vi "Run Process.vi"(8 "error in":errorcluster, 9 "Processes":cluster{"VI":refnum<vi>, "Parameters":variant}[](array[cluster]), 11 "VS Plugin Inline Async API in":refnum<class "VS Plugin Inline Async API.lvclass">) -> (0 "error out":errorcluster, 3 "VS Plugin Inline Async API out":refnum<class "VS Plugin Inline Async API.lvclass">)   [LabVIEW 2024, in "VS Plugin Inline Async API.lvlib" / "VS Plugin Inline Async API.lvclass"]
uses:
  VS Plugin Inline Async API.lvclass
  VS Plugin Inline Async API.lvclass/VS Plugin Inline Async API.ctl
  Process/Process.lvclass
  Process/Process.lvclass/Process.ctl
  Process/Write Name.vi
  Process/Write Process.Stop.vi
  Process/Write Process.Trigger.vi
  Process/Write Data Access.vi
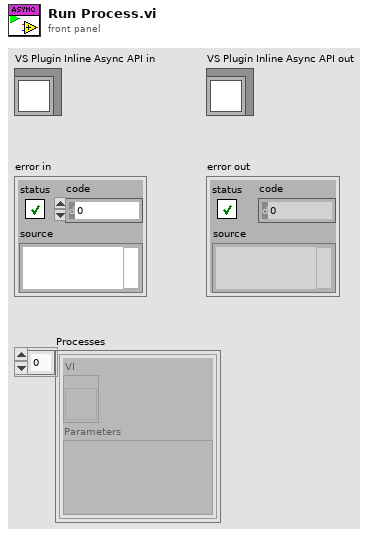
[diagram p1: front panel]
types:
  T1 = cluster{"read mode":enum16{"polling", "blocking"}, "write mode":enum16{"polling", "blocking"}}
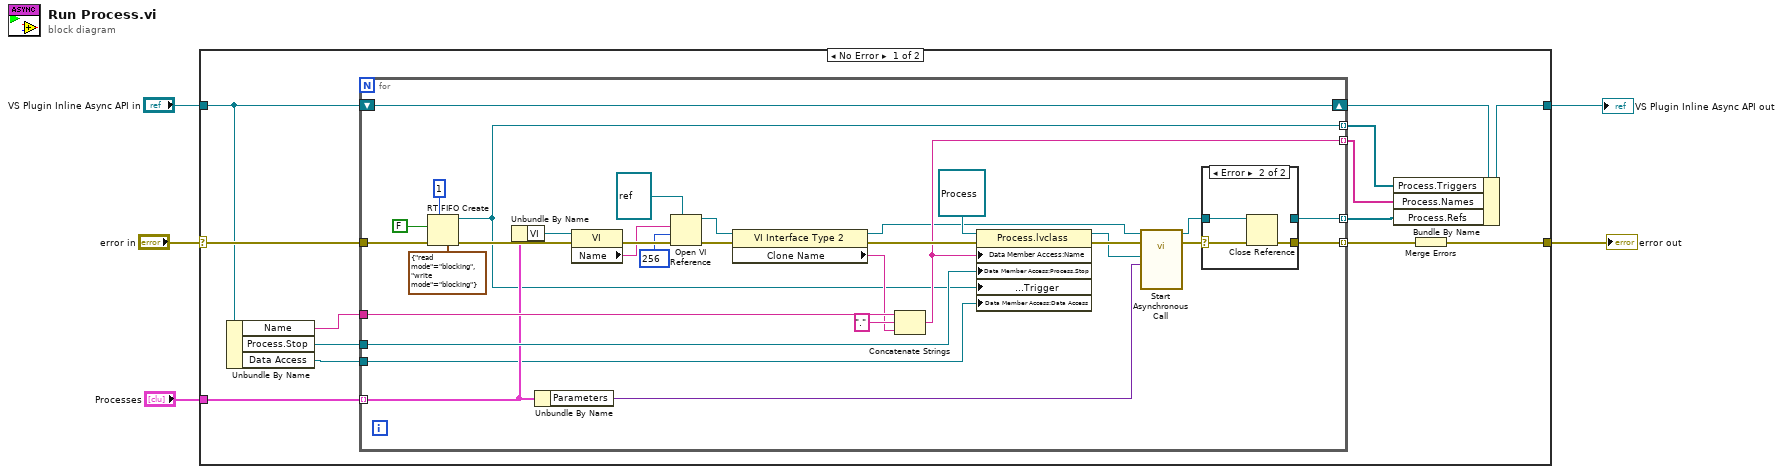
[diagram p0: block diagram]
diagram:
  n1 = case shown="No Error" "error in" {
    selector: "error in" -> [w18 w56]
    tunnel: [w17 w56] -> w4
    tunnel: "Processes" -> [w15 _]
    tunnel: "VS Plugin Inline Async API in" -> [w11 w55]
    tunnel: [w12 w55] -> w1
    frame No Error {
      n2 = Unbundle By Name(w11) -> ("Name"=w10:string, "Process.Stop"=w9:refnum<data-value>, "Data Access"=w7:refnum<class "Plugin Data Access Engine.lvclass">)
      n3 = for {
        tunnel: [w49] -> w16 mode=indexing
        tunnel: [w41] -> w14 mode=indexing
        tunnel: w18 -> [w43]
        tunnel: w15 -> [w29] mode=indexing
        shift-right: [w38] -> w13
        shift-left: w11 -> [w38]
        tunnel: w10 -> [w37]
        tunnel: w9 -> [w33]
        tunnel: [w31] -> w8 mode=indexing
        tunnel: w7 -> [w27]
        tunnel: [w19] -> w6 mode=indexing
        n4 = RT FIFO Create(1:FALSE, 3:w43, 4:u32 1 ("size (10)"), 7:T1 {"read mode"=enum."blocking", "write mode"=enum."blocking"} ("r/w modes (polling,polling)")) -> (8:w19:refnum<k33>, 11:w42:errorcluster)  [unwired: 4 in, 1 out]
        n5 = Unbundle By Name(w29) -> ("VI"=w30:refnum<vi>)
        n6 = Unbundle By Name(w29) -> ("Parameters"=w28:variant)
        n7 = property class="VI"(reference=w30, error in=w42) -> (error out=w45:errorcluster, "Name"=w36:string)  [unwired: 1 out]
        n8 = Open VI Reference(type specifier VI Refnum (for type only)=refnum<vi> refnum, vi path=w36, options=256, error in (no error)=w45) -> (vi reference=w26:refnum<vi>, error out=w47:errorcluster)  [unwired: 2 out]
        n9 = property class="VI Interface Type 2"(reference=w26, error in=w47) -> (reference out=w25:refnum<vi>, error out=w46:errorcluster, "Clone Name"=w24:string)
        n10 = Concatenate Strings(w37, "." ("string"), w24) -> (w31:string)
        n11 = property class="Process.lvclass"(reference=refnum<class "Process.lvclass"> refnum ("FPGA Addon Engine.lvlib:Process.lvclass"), error in=w46, "Data Member Access:Name"=w31, "Data Member Access:Process.Stop"=w33, "Data Member Access:Process.Trigger"=w19, "Data Member Access:Data Access"=w27) -> (reference out=w32:refnum<class "Process.lvclass">, error out=w44:errorcluster)
        n12 = call-by-ref "Start Asynchronous Call"(reference=w25, error in=w44, "Parameters"=w28, "Process"=w32) -> (reference out=w40:refnum<vi>, error out=w48:errorcluster)  [unwired: 10 in]
        n13 = case shown="Error" w48 {
          selector: w48 -> [w51 w54]
          tunnel: w40 -> [w50 w52]
          tunnel: [w51 w53] -> w49
          tunnel: [w50 _] -> w41
          frame No Error {
          }
          frame Error {
            n14 = Close Reference(reference=w52, error in (no error)=w54) -> (error out=w53:errorcluster)
          }
        }
      }
      n15 = Bundle By Name(cluster=w13, "Process.Triggers"=w6, "Process.Names"=w8, "Process.Refs"=w14) -> (w12:refnum<class "VS Plugin Inline Async API.lvclass">)
      n16 = Merge Errors(w16) -> (w17:errorcluster)
    }
    frame Error {
    }
  }
  "error out" <- w4
  "VS Plugin Inline Async API out" <- w1
